vi "AdaBoostClassifier.vi"(8 "error in":errorcluster) -> (0 "error out":errorcluster, 3 "out":refnum<class "AdaBoostClassifier.lvclass">)   [LabVIEW 2020]
doc: "An AdaBoost classifier.\n\n An AdaBoost [1] classifier is a meta-estimator that begins by fitting a\n classifier on the original dataset and then fits additional copies of the\n classifier on the same dataset but where the weights of incorrectly\n classified instances are adjusted such that subsequent classifiers focus\n more on difficult cases.\n\n This class implements the algorithm known as AdaBoost-SAMME [2].\n\n Read more in the :ref:`User Guide <adaboost>`.\n\n .. versionadded:: 0.14\n\n Parameters\n ----------\n base_estimator : object, default=None\n The base estimator from which the boosted ensemble is built.\n Support for sample weighting is required, as well as proper\n ``classes_`` and ``n_classes_`` attributes. If ``None``, then\n the base estimator is :class:`~sklearn.tree.DecisionTreeClassifier`\n initialized with `max_depth=1`.\n\n n_estimators : int, default=50\n The maximum number of estimators at which boosting is terminated.\n In case of perfect fit, the learning procedure is stopped early.\n\n learning_rate : float, default=1.\n Weight applied to each classifier at each boosting iteration. A higher\n learning rate increases the contribution of each classifier. There is\n a trade-off between the `learning_rate` and `n_estimators` parameters.\n\n algorithm : {'SAMME', 'SAMME.R'}, default='SAMME.R'\n If 'SAMME.R' then use the SAMME.R real boosting algorithm.\n ``base_estimator`` must support calculation of class probabilities.\n If 'SAMME' then use the SAMME discrete boosting algorithm.\n The SAMME.R algorithm typically converges faster than SAMME,\n achieving a lower test error with fewer boosting iterations.\n\n random_state : int, RandomState instance or None, default=None\n Controls the random seed given at each `base_estimator` at each\n boosting iteration.\n Thus, it is only used when `base_estimator` exposes a `random_state`.\n Pass an int for reproducible output across multiple function calls.\n See :term:`Glossary <random_state>`.\n\n Attributes\n ----------\n base_estimator_ : estimator\n The base estimator from which the ensemble is grown.\n\n estimators_ : list of classifiers\n The collection of fitted sub-estimators.\n\n classes_ : ndarray of shape (n_classes,)\n The classes labels.\n\n n_classes_ : int\n The number of classes.\n\n estimator_weights_ : ndarray of floats\n Weights for each estimator in the boosted ensemble.\n\n estimator_errors_ : ndarray of floats\n Classification error for each estimator in the boosted\n ensemble.\n\n feature_importances_ : ndarray of shape (n_features,)\n The impurity-based feature importances if supported by the\n ``base_estimator`` (when based on decision trees).\n\n Warning: impurity-based feature importances can be misleading for\n high cardinality features (many unique values). See\n :func:`sklearn.inspection.permutation_importance` as an alternative.\n\n See Also\n --------\n AdaBoostRegressor : An AdaBoost regressor that begins by fitting a\n regressor on the original dataset and then fits additional copies of\n the regressor on the same dataset but where the weights of instances\n are adjusted according to the error of the current prediction.\n\n GradientBoostingClassifier : GB builds an additive model in a forward\n stage-wise fashion. Regression trees are fit on the negative gradient\n of the binomial or multinomial deviance loss function. Binary\n classification is a special case where only a single regression tree is\n induced.\n\n sklearn.tree.DecisionTreeClassifier : A non-parametric supervised learning\n method used for classification.\n Creates a model that predicts the value of a target variable by\n learning simple decision rules inferred from the data features.\n\n References\n ----------\n .. [1] Y. Freund, R. Schapire, \"A Decision-Theoretic Generalization of\n on-Line Learning and an Application to Boosting\", 1995.\n\n .. [2] J. Zhu, H. Zou, S. Rosset, T. Hastie, \"Multi-class AdaBoost\", 2009.\n\n \nAvailable methods:\nPredict Log Proba\nPredict Proba\nFit\nPredict\nScore\nGet Attributes\nGet Params\nSet Params"
uses:
  AdaBoostClassifier.lvclass
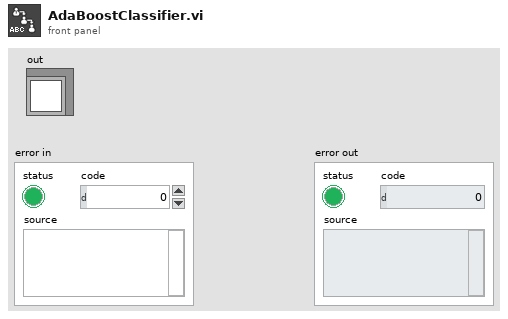
[diagram p1: front panel]
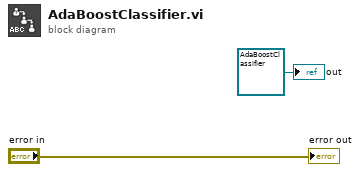
[diagram p0: block diagram]
diagram:
  "out" <- refnum<class "AdaBoostClassifier.lvclass"> refnum ("model")
  "error out" <- "error in"
